vi "Quit Program.vi"(8 "error in (no error)":errorcluster) -> ()   [LabVIEW 2020, in "Architecture Support.lvlib"]
uses:
  Architecture Support.lvlib
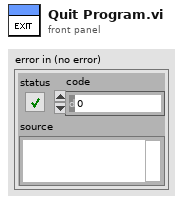
[diagram p1: front panel]
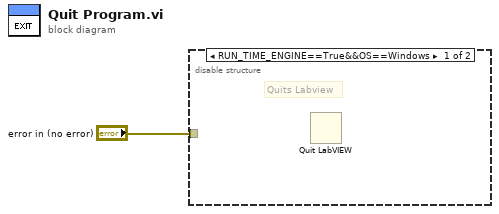
[diagram p0: block diagram]
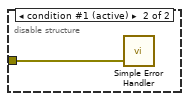
[diagram p2: hidden frame]
diagram:
  n1 = disable-structure shown="RUN_TIME_ENGINE==True&&OS==Windows" {
    disable-tunnel: "error in (no error)" -> [_ w2]
    frame condition #0 {
      # "Quits Labview"
      n2 = Quit LabVIEW() -> ()  [unwired: 1 in]
    }
    frame condition #1 (active) {
      n3 = call <vilib>:"Simple Error Handler.vi"("error in (no error)"=w2) -> ()  [unwired: 4 in, 5 out]
    }
  }
